vi "SPX Fit cooling curve.vi"(6 "Resistances":dbl[](array[numeric]), 8 "Time":dbl[](array[numeric]), 9 "Radj":dbl step=0.01, 10 "cold R":dbl) -> (1 "error":dbl format="%#_6f", 2 "Zero R":dbl, 3 "Stator":cluster{dbl[], dbl[]}[](graph))   [LabVIEW 2017]
uses:
  <vilib>/Analysis/NI_AALPro.lvlib
panel:
  out "Waveform Graph":dbl[](graph)
  out "Array":dbl[](array[numeric])
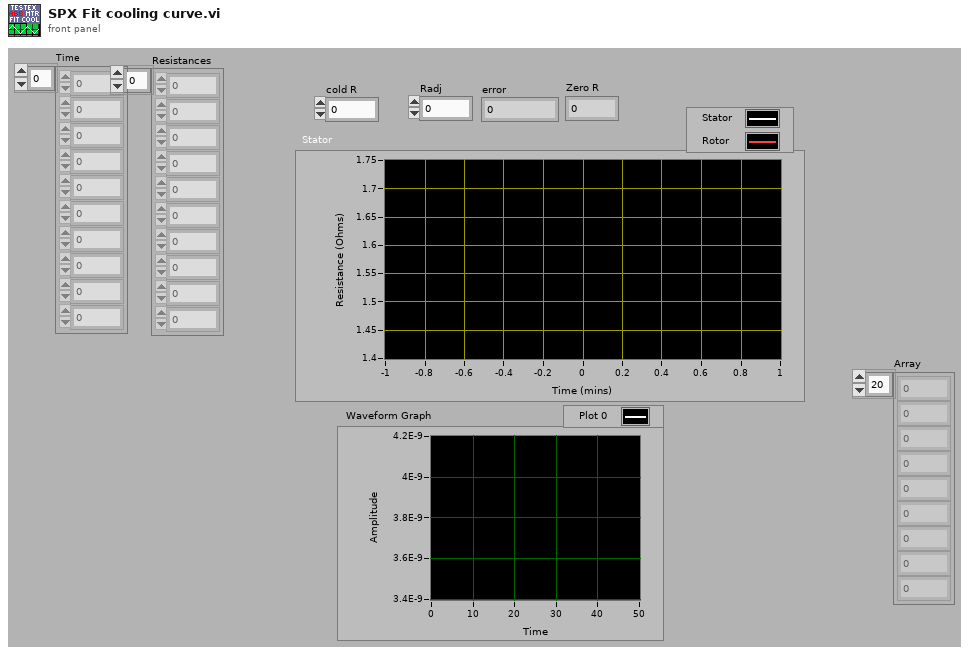
[diagram p1: front panel]
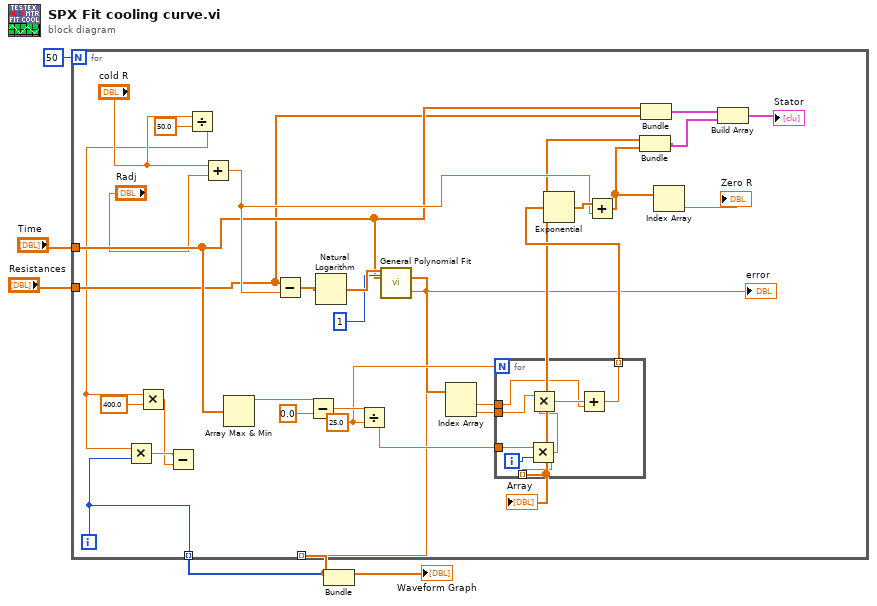
[diagram p0: block diagram]
diagram:
  n1 = for {
    N: 50 -> [_]
    tunnel: "Time" -> [w13]
    tunnel: "Resistances" -> [w12]
    tunnel: [w6] -> w2 mode=indexing
    tunnel: [w7] -> w1 mode=indexing
    i -> [w6]
    w24 = 25.0 ("y")
    n2 = Divide(x="cold R", y=50.0) -> (x/y=w11:dbl)
    n3 = Multiply(x=w11, y=w6) -> (x*y=w14:dbl)
    n4 = Multiply(x=w11, y=400.0) -> (x*y=w9:dbl)
    n5 = Subtract(x=w14, y=w9) -> ()  [unwired: 1 out]
    n6 = Add(x="cold R", y="Radj") -> (x+y=w32:dbl)
    n7 = Array Max & Min(array=w13) -> (max value=w26:dbl)  [unwired: 3 out]
    n8 = Subtract(x=w12, y=w32) -> (x-y=w36:dbl[])
    n9 = Subtract(x=w26, y=0.0) -> (x-y=w25:dbl)
    n10 = Natural Logarithm(1:w36) -> (0:w28:dbl[])
    n11 = Divide(x=w25, y=w24) -> (x/y=w23:dbl)
    n12 = call <vilib>:"General Polynomial Fit.vi"("Y"=w28, "polynomial order"=1, "X"=w13) -> ("Polynomial Coefficients"=w22:dbl[], "residue"=w7:dbl)  [unwired: 9 in, 2 out]
    "error" <- w7
    n13 = Index Array(array=w22) -> (element #1=w19:dbl, element #2=w18:dbl)  [unwired: 2 in]
    n14 = for {
      N: w24 -> [_]
      tunnel: w23 -> [w40]
      tunnel: w19 -> [w37]
      tunnel: [w41] -> w20 mode=indexing
      tunnel: [w39] -> w17 mode=indexing
      tunnel: w18 -> [w38]
      i -> [w43]
      n15 = Multiply(x=w40, y=w43) -> (x*y=w39:dbl)
      n16 = Multiply(x=w38, y=w39) -> (x*y=w42:dbl)
      n17 = Add(x=w42, y=w37) -> (x+y=w41:dbl)
    }
    "Array" <- w17
    n18 = Exponential(1:w20) -> (0:w34:dbl[])
    n19 = Add(x=w34, y=w32) -> (x+y=w30:dbl[])
    n20 = Bundle(w17, w30) -> (w31:cluster{dbl[], dbl[]})  [unwired: 1 in]
    n21 = Bundle("Time"=w13, "Resistances"=w12) -> (w35:cluster{"Time":dbl[], "Resistances":dbl[]})  [unwired: 1 in]
    n22 = Index Array(array=w30) -> (element=→"Zero R":dbl)  [unwired: 1 in]
    n23 = Build Array(w35, w31) -> (→"Stator":cluster{"Time":dbl[], "Resistances":dbl[]}[])
  }
  "Waveform Graph" <- w1
  n24 = Bundle(w2, w1) -> ()  [unwired: 1 in, 1 out]
